vi "getPhase.vi"(8 "error in (no error)":errorcluster, 11 "SingleTone.lvclass in":refnum<class "SingleTone.lvclass">) -> (0 "error out":errorcluster, 2 "phase":dbl, 3 "SingleTone.lvclass out":refnum<class "SingleTone.lvclass">)   [LabVIEW 2011, in "Tools.lvlib" / "Scripting.lvlib" / "SingleTone.lvclass"]
uses:
  SingleTone.lvclass
  SingleTone.lvclass/SingleTone.ctl
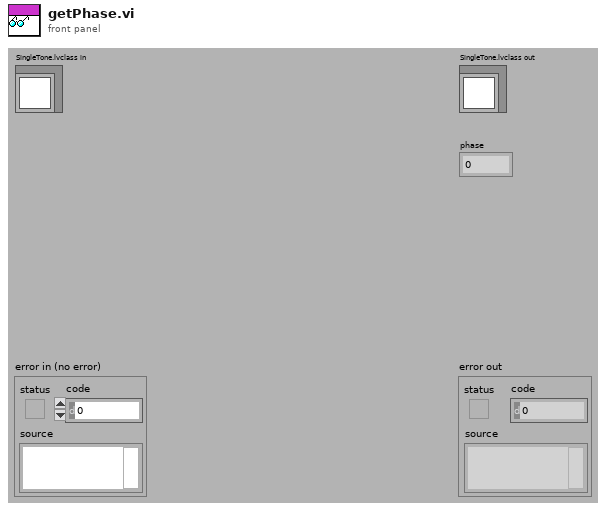
[diagram p1: front panel]
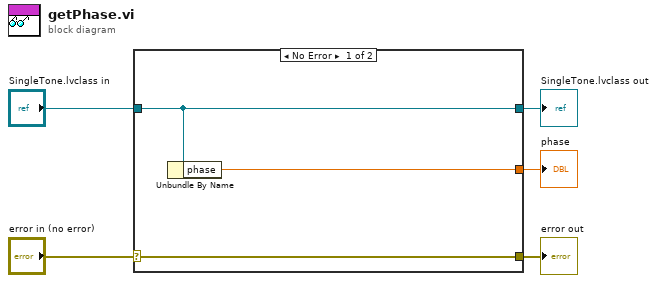
[diagram p0: block diagram]
diagram:
  n1 = case shown="No Error" "error in (no error)" {
    selector: "error in (no error)" -> [w8 w9]
    tunnel: [w8 w9] -> w4
    tunnel: [w7 w10] -> w2
    tunnel: "SingleTone.lvclass in" -> [w7 w10]
    tunnel: [w6 _] -> w1
    frame No Error {
      n2 = Unbundle By Name(w7) -> ("phase"=w6:dbl)
    }
    frame Error {
    }
  }
  "error out" <- w4
  "SingleTone.lvclass out" <- w2
  "phase" <- w1
